vi "send_SQMS_msg.vi"(5 "alarm_interval":dbl=300.0, 6 "msg":string, 7 "enabled":bool=TRUE, 8 "time_last_alarm_in":timestamp, 9 "title":string="SQMS Message", 10 "warning":bool, 11 "error":bool) -> (0 "time_last_alarm_out":timestamp, 3 "alarm_status":u32(colorbox), 4 "msg_status":bool)   [LabVIEW 2019]
panel:
  in  "to":string="Discord/TargetAlarm"
  out "full_message":string
  out "resp2":string
  out "resp1":string
  out "resp3":string
  in  "timeout":i32=1000
  in  "port":u16=11111
  in  "address":string="192.168.24.72"
  # "\"time_..._in\" and \"time_..._out\" must be connected\n via Feedback Node or Shift Register in a loop that calls this sub VI."
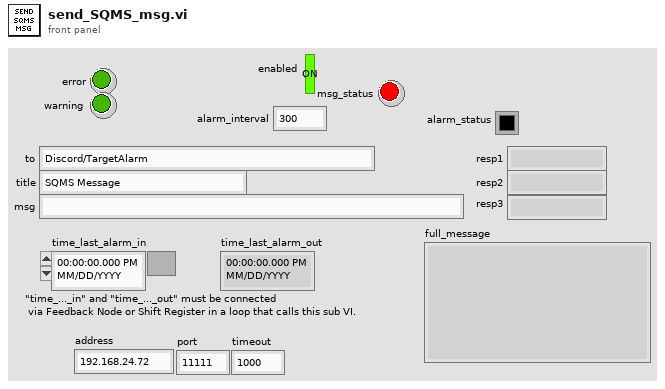
[diagram p1: front panel]
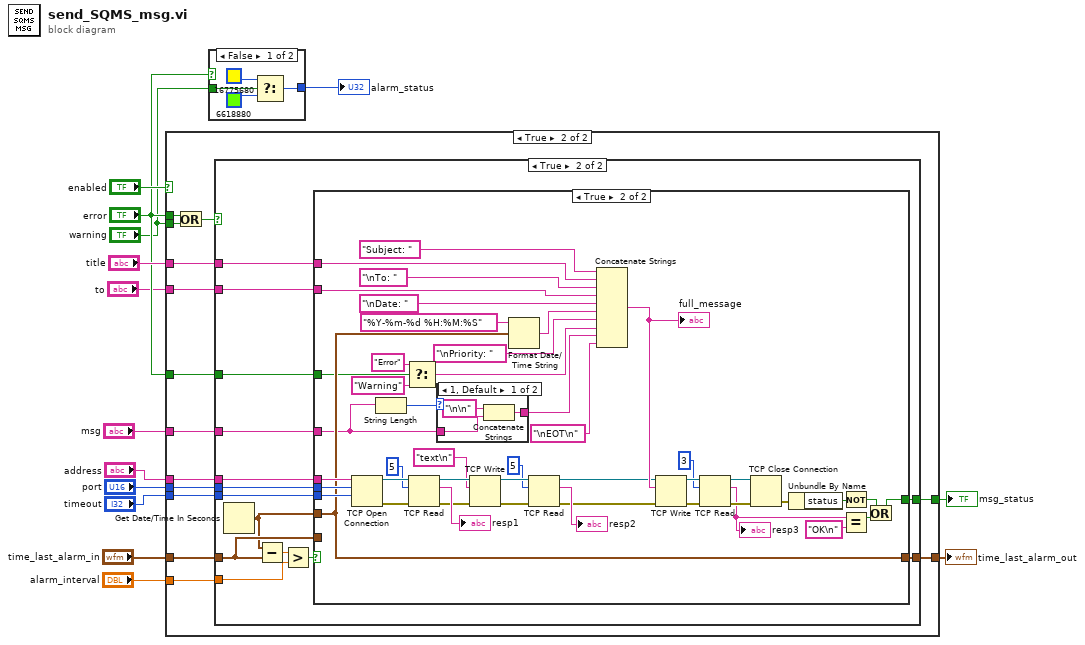
[diagram p0: block diagram]
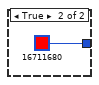
[diagram p2: hidden frame]
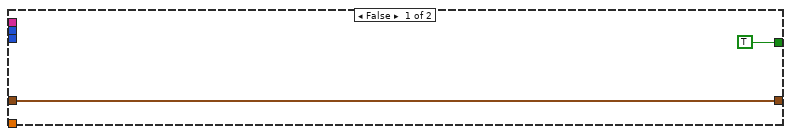
[diagram p3: hidden frame]
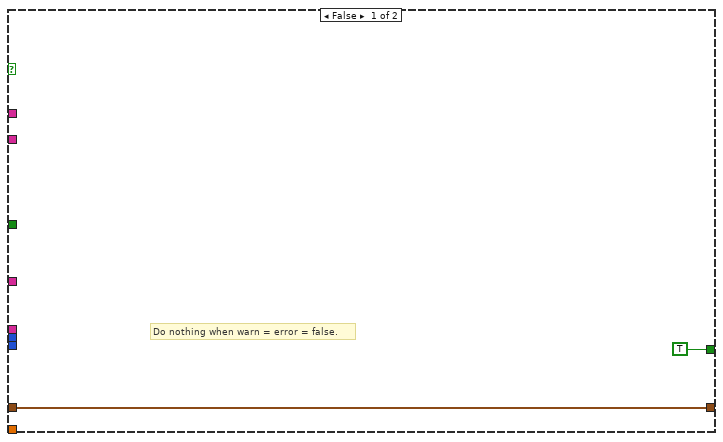
[diagram p4: hidden frame]
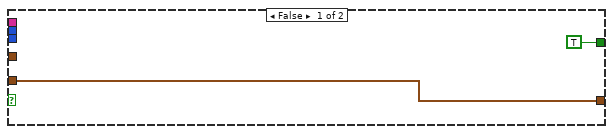
[diagram p5: hidden frame]
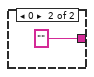
[diagram p6: hidden frame]
diagram:
  n1 = case shown="True" "enabled" {
    tunnel: "error" -> [_ w30]
    tunnel: "warning" -> [_ w29]
    tunnel: [w16 w27] -> w13
    tunnel: "time_last_alarm_in" -> [w16 w26]
    tunnel: "alarm_interval" -> [_ w25]
    tunnel: "address" -> [_ w24]
    tunnel: "port" -> [_ w23]
    tunnel: "timeout" -> [_ w22]
    tunnel: "title" -> [_ w21]
    tunnel: "error" -> [_ w20]
    tunnel: [TRUE w19] -> w6
    tunnel: "msg" -> [_ w18]
    tunnel: "to" -> [_ w17]
    frame False {
    }
    frame True {
      n2 = Or(x=w30, y=w29) -> (x .or. y?=w28:bool)
      n3 = case shown="True" w28 {
        tunnel: [w32 w43] -> w27
        tunnel: w26 -> [w32 w42]
        tunnel: w25 -> [_ w45]
        tunnel: w24 -> [_ w40]
        tunnel: w23 -> [_ w39]
        tunnel: w22 -> [_ w38]
        tunnel: w21 -> [_ w37]
        tunnel: w20 -> [_ w36]
        tunnel: [TRUE w35] -> w19
        tunnel: w18 -> [_ w34]
        tunnel: w17 -> [_ w33]
        frame False {
          # "Do nothing when warn = error = false."
        }
        frame True {
          n4 = Get Date/Time In Seconds() -> (seconds since 1Jan1904=w41:timestamp)
          n5 = Subtract(x=w41, y=w42) -> (x-y=w46:dbl)
          n6 = Greater?(x=w46, y=w45) -> (0:w44:bool)
          n7 = case shown="True" w44 {
            tunnel: [w48 w86] -> w43
            tunnel: w42 -> [w48 _]
            tunnel: w41 -> [_ w86]
            tunnel: w40 -> [_ w94]
            tunnel: w39 -> [_ w93]
            tunnel: w38 -> [_ w92]
            tunnel: w37 -> [_ w89]
            tunnel: w36 -> [_ w78]
            tunnel: [TRUE w55] -> w35
            tunnel: w34 -> [_ w51]
            tunnel: w33 -> [_ w49]
            frame False {
            }
            frame True {
              n8 = TCP Open Connection(address=w94, remote port or service name=w93, timeout ms (60000)=w92) -> (connection ID=w91:refnum<k5>, error out=w65:errorcluster)  [unwired: 2 in]
              n9 = String Length(string=w51) -> (length=w53:i32)
              n10 = Select(t="Error", s=w78, f="Warning") -> (s? t:f=w76:string)
              n11 = TCP Read(connection ID=w91, bytes to read=5, error in (no error)=w65) -> (connection ID out=w73:refnum<k5>, data out=→"resp1":string, error out=w64:errorcluster)  [unwired: 2 in]
              n12 = case shown="1, Default" w53 {
                tunnel: [w97 ""] -> w52
                tunnel: w51 -> [w95 _]
                frame 1, Default {
                  n13 = Concatenate Strings("\n\n" ("string"), w95) -> (w97:string)
                }
                frame 0 {
                }
              }
              n14 = TCP Write(connection ID=w73, data in="text\n", error in (no error)=w64) -> (connection ID out=w70:refnum<k5>, error out=w63:errorcluster)  [unwired: 1 in, 1 out]
              n15 = Format Date/Time String(time format string (%c)="%Y-%m-%d %H:%M:%S", seconds (now)=w86) -> (date/time string=w85:string)  [unwired: 1 in]
              n16 = TCP Read(connection ID=w70, bytes to read=5, error in (no error)=w63) -> (connection ID out=w68:refnum<k5>, data out=→"resp2":string, error out=w62:errorcluster)  [unwired: 2 in]
              n17 = Concatenate Strings("Subject: ", w89, "\nTo: ", w49, "\nDate: ", w85, "\nPriority: ", w76, w52, "\nEOT\n") -> (w83:string)
              "full_message" <- w83
              n18 = TCP Write(connection ID=w68, data in=w83, error in (no error)=w62) -> (connection ID out=w82:refnum<k5>, error out=w81:errorcluster)  [unwired: 1 in, 1 out]
              n19 = TCP Read(connection ID=w82, bytes to read=3, error in (no error)=w81) -> (connection ID out=w79:refnum<k5>, data out=w59:string, error out=w80:errorcluster)  [unwired: 2 in]
              "resp3" <- w59
              n20 = TCP Close Connection(connection ID=w79, error in (no error)=w80) -> (error out=w61:errorcluster)  [unwired: 1 in, 1 out]
              n21 = Unbundle By Name(w61) -> ("status"=w60:bool)
              n22 = Not(x=w60) -> (.not. x?=w56:bool)
              n23 = Equal?(x=w59, y="OK\n") -> (x = y?=w57:bool)
              n24 = Or(x=w56, y=w57) -> (x .or. y?=w55:bool)
            }
          }
        }
      }
    }
  }
  "time_last_alarm_out" <- w13
  "msg_status" <- w6
  n25 = case shown="False" "error" {
    tunnel: "warning" -> [w102 _]
    tunnel: [w99 u32 16711680 ("alarm_status")] -> w2
    frame False {
      n26 = Select(t=u32 16775680 ("alarm_status"), s=w102, f=u32 6618880 ("alarm_status")) -> (s? t:f=w99:u32)
    }
    frame True {
    }
  }
  "alarm_status" <- w2
